vi "Script Msg Msg VI.vi"(4 "Name":string, 6 "Name Msg Refs.Msg VI":refnum<vi>, 8 "error in":errorcluster, 9 "Msg Output Terminal Map":T1, 10 "Msg Terminal Map":T3) -> (0 "error out":errorcluster)   [LabVIEW 2025, in "_Msg Rescript.lvlib" / "_Msg Rescript.lvclass"]
uses:
  _Msg Rescript.lvclass
  _Msg Rescript.lvclass/_Msg Rescript.ctl
  <vilib>/Utility/traverseref.llb/TRef TravTarget.ctl
  Msg Terminal Attributes.ctl
  Msg Terminal Map.ctl
  Msg Output Terminal Attributes.ctl
  Msg Output Terminal Map.ctl
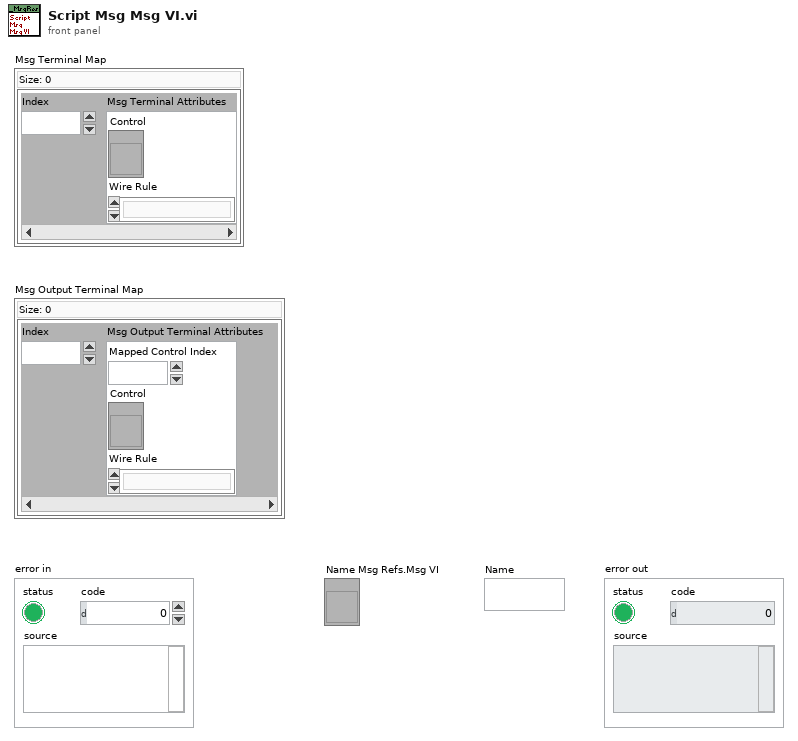
[diagram p1: front panel]
types:
  T1 = typedef "_Msg Rescript.lvlib/_Msg Rescript.lvclass/Msg Output Terminal Map.ctl" = map{i32, T2}
  T2 = typedef "_Msg Rescript.lvlib/_Msg Rescript.lvclass/Msg Output Terminal Attributes.ctl" = cluster{"Mapped Control Index":i32, "Control":refnum<vi>, "Wire Rule":enum16{"Invalid Wire Rule", "Required", "Recommended", "Optional", "Dynamic Dispatch"}}
  T3 = typedef "_Msg Rescript.lvlib/_Msg Rescript.lvclass/Msg Terminal Map.ctl" = map{i32, T4}
  T4 = typedef "_Msg Rescript.lvlib/_Msg Rescript.lvclass/Msg Terminal Attributes.ctl" = cluster{"Control":refnum<vi>, "Wire Rule":enum16{"Invalid Wire Rule", "Required", "Recommended", "Optional", "Dynamic Dispatch"}}
  T5 = typedef "TRef TravTarget.ctl" = enum16{"FP", "BD", "Other"}
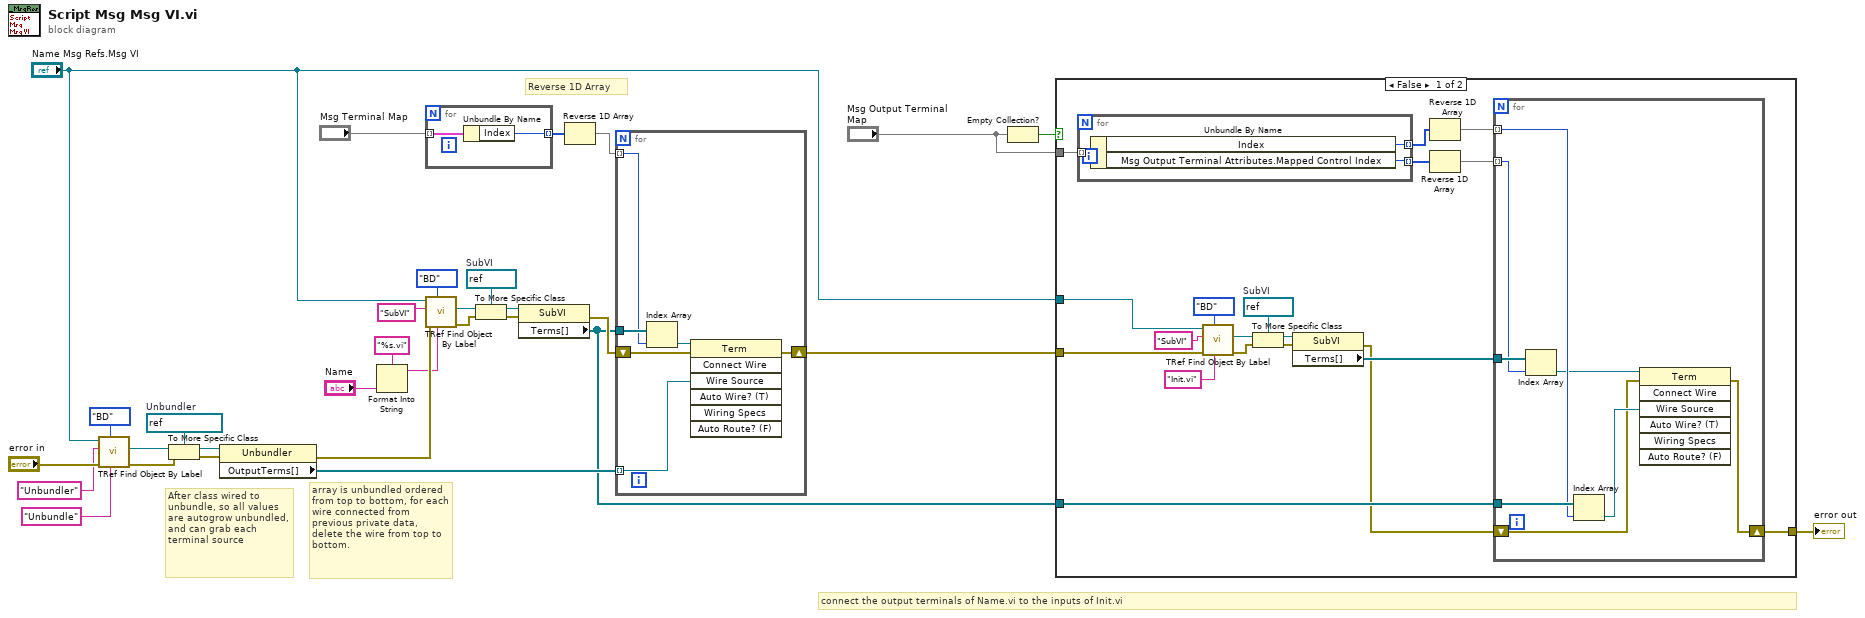
[diagram p0: block diagram]
diagram:
  w16 = refnum<vi> refnum  # Unbundler
  w30 = refnum<vi> refnum  # SubVI
  # "connect the output terminals of Name.vi to the inputs of Init.vi"
  # "Reverse 1D Array"
  # "array is unbundled ordered from top to bottom, for each wire connected from previous private data, delete the wire from top to bottom."
  # "After class wired to unbundle, so all values are autogrow unbundled, and can grab each terminal source"
  n1 = call <vilib>:"TRef Find Object By Label.vi"("Label"="Unbundle", "Traverse Target"=TRef_TravTarget."BD", "error in (no error)"="error in", "Class Name"="Unbundler", "VI Ref"="Name Msg Refs.Msg VI") -> ("error out"=w17:errorcluster, "Found Obj Ref"=w15:refnum<vi>)  [unwired: 3 in, 2 out]
  n2 = To More Specific Class(target class=w16, reference=w15, error in=w17) -> (specific class reference=w12:refnum<vi>, error out=w9:errorcluster)
  n3 = property class="Unbundler"(reference=w12, error in=w9) -> (error out=w21:errorcluster, "OutputTerms[]"=w8:refnum<vi>[])  [unwired: 1 out]
  n4 = Format Into String(format string="%s.vi", "Name") -> (resulting string=w18:string)  [unwired: 2 in, 1 out]
  n5 = for {
    tunnel: "Msg Terminal Map" -> [w33] mode=indexing
    tunnel: [w32] -> w25 mode=indexing
    n6 = Unbundle By Name(w33) -> ("Index"=w32:i32)
  }
  n7 = call <vilib>:"TRef Find Object By Label.vi"("Label"=w18, "Traverse Target"=TRef_TravTarget."BD", "error in (no error)"=w21, "Class Name"="SubVI", "VI Ref"="Name Msg Refs.Msg VI") -> ("error out"=w29:errorcluster, "Found Obj Ref"=w20:refnum<vi>)  [unwired: 3 in, 2 out]
  n8 = To More Specific Class(target class=w30, reference=w20, error in=w29) -> (specific class reference=w27:refnum<vi>, error out=w26:errorcluster)
  n9 = property class="SubVI"(reference=w27, error in=w26) -> (error out=w24:errorcluster, "Terms[]"=w4:refnum<vi>[])  [unwired: 1 out]
  n10 = Reverse 1D Array(array=w25) -> (reversed array=w22:i32[])
  n11 = for {
    tunnel: w4 -> [w39]
    tunnel: w22 -> [w38] mode=indexing
    shift-right: [w35] -> w1
    shift-left: w24 -> [w36]
    tunnel: w8 -> [w34] mode=indexing
    n12 = Index Array(array=w39, index=w38) -> (element=w37:refnum<vi>)
    n13 = invoke class="Term" method="Connect Wire"(reference=w37, error in=w36, "Wire Source"=w34) -> (error out=w35:errorcluster)  [unwired: 4 in, 6 out]
  }
  n14 = Empty Collection?(1:"Msg Output Terminal Map") -> (0:w6:bool)
  n15 = case shown="False" w6 {
    tunnel: "Msg Output Terminal Map" -> [w57 _]
    tunnel: w4 -> [w55 _]
    tunnel: [w52 w70] -> w3
    tunnel: "Name Msg Refs.Msg VI" -> [w44 _]
    tunnel: w1 -> [w42 w70]
    frame False {
      w50 = refnum<vi> refnum  # SubVI
      n16 = for {
        tunnel: w57 -> [w61] mode=indexing
        tunnel: [w60] -> w58 mode=indexing
        tunnel: [w59] -> w56 mode=indexing
        n17 = Unbundle By Name(w61) -> ("Index"=w60:i32, "Msg Output Terminal Attributes.Mapped Control Index"=w59:i32)
      }
      n18 = call <vilib>:"TRef Find Object By Label.vi"("Label"="Init.vi", "Traverse Target"=TRef_TravTarget."BD", "error in (no error)"=w42, "Class Name"="SubVI", "VI Ref"=w44) -> ("error out"=w49:errorcluster, "Found Obj Ref"=w46:refnum<vi>)  [unwired: 3 in, 2 out]
      n19 = To More Specific Class(target class=w50, reference=w46, error in=w49) -> (specific class reference=w48:refnum<vi>, error out=w47:errorcluster)
      n20 = property class="SubVI"(reference=w48, error in=w47) -> (error out=w41:errorcluster, "Terms[]"=w43:refnum<vi>[])  [unwired: 1 out]
      n21 = Reverse 1D Array(array=w58) -> (reversed array=w53:i32[])
      n22 = Reverse 1D Array(array=w56) -> (reversed array=w54:i32[])
      n23 = for {
        tunnel: w43 -> [w69]
        tunnel: w55 -> [w68]
        tunnel: w54 -> [w67] mode=indexing
        tunnel: w53 -> [w66] mode=indexing
        shift-right: [w62] -> w52
        shift-left: w41 -> [w63]
        n24 = Index Array(array=w69, index=w67) -> (element=w65:refnum<vi>)
        n25 = Index Array(array=w68, index=w66) -> (element=w64:refnum<vi>)
        n26 = invoke class="Term" method="Connect Wire"(reference=w65, error in=w63, "Wire Source"=w64) -> (error out=w62:errorcluster)  [unwired: 4 in, 6 out]
      }
    }
    frame True {
    }
  }
  "error out" <- w3
